vi "LDA_IP.vi"() -> (0 "error out":errorcluster)   [LabVIEW 2022 SP3]
uses:
  Globals/Meas_global.vi
  Globals/LDA_global.vi
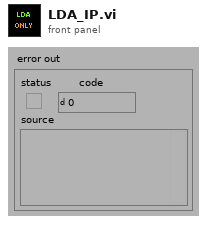
[diagram p1: front panel]
types:
  T1 = typedef "Setup.ctl" = enum16{"Run Program", "Show Setup", "Save Current Setup", "Setup Front Panel"}
  T2 = typedef "LDA_Channel.ctl" = cluster{"Wavelength (nm)":dbl, "Vel Comp":string, "Max Velocity":dbl, "Min Velocity":dbl, "Max Record length":u16, "Signal gain (dB)":i16, "High voltage":i16, "Optics Conversion Factor":dbl, "Min Record length":u16, "Multiply Velocity by -1":bool, "Signal to Noise Ratio":string, "Validation Ratio":string, "Probe":string, "Laser":string, "BSA":string, "Lense":string, "Beam Separation (mm)":dbl, "Focal Length (mm)":dbl, "COLOUR":u32, "BSA IP":string, "Velocity Range (m/s)":dbl, "Centre Velocity (m/s)":dbl, "Unshifted mW":dbl, "Shifted mW":dbl, "Bandwidth Hz":dbl, "Req Sampling Rate Hz":dbl, "Ch":i32, "CenterFreq Hz":dbl, "Laser IP":string, "Sync Delay (s)":dbl}
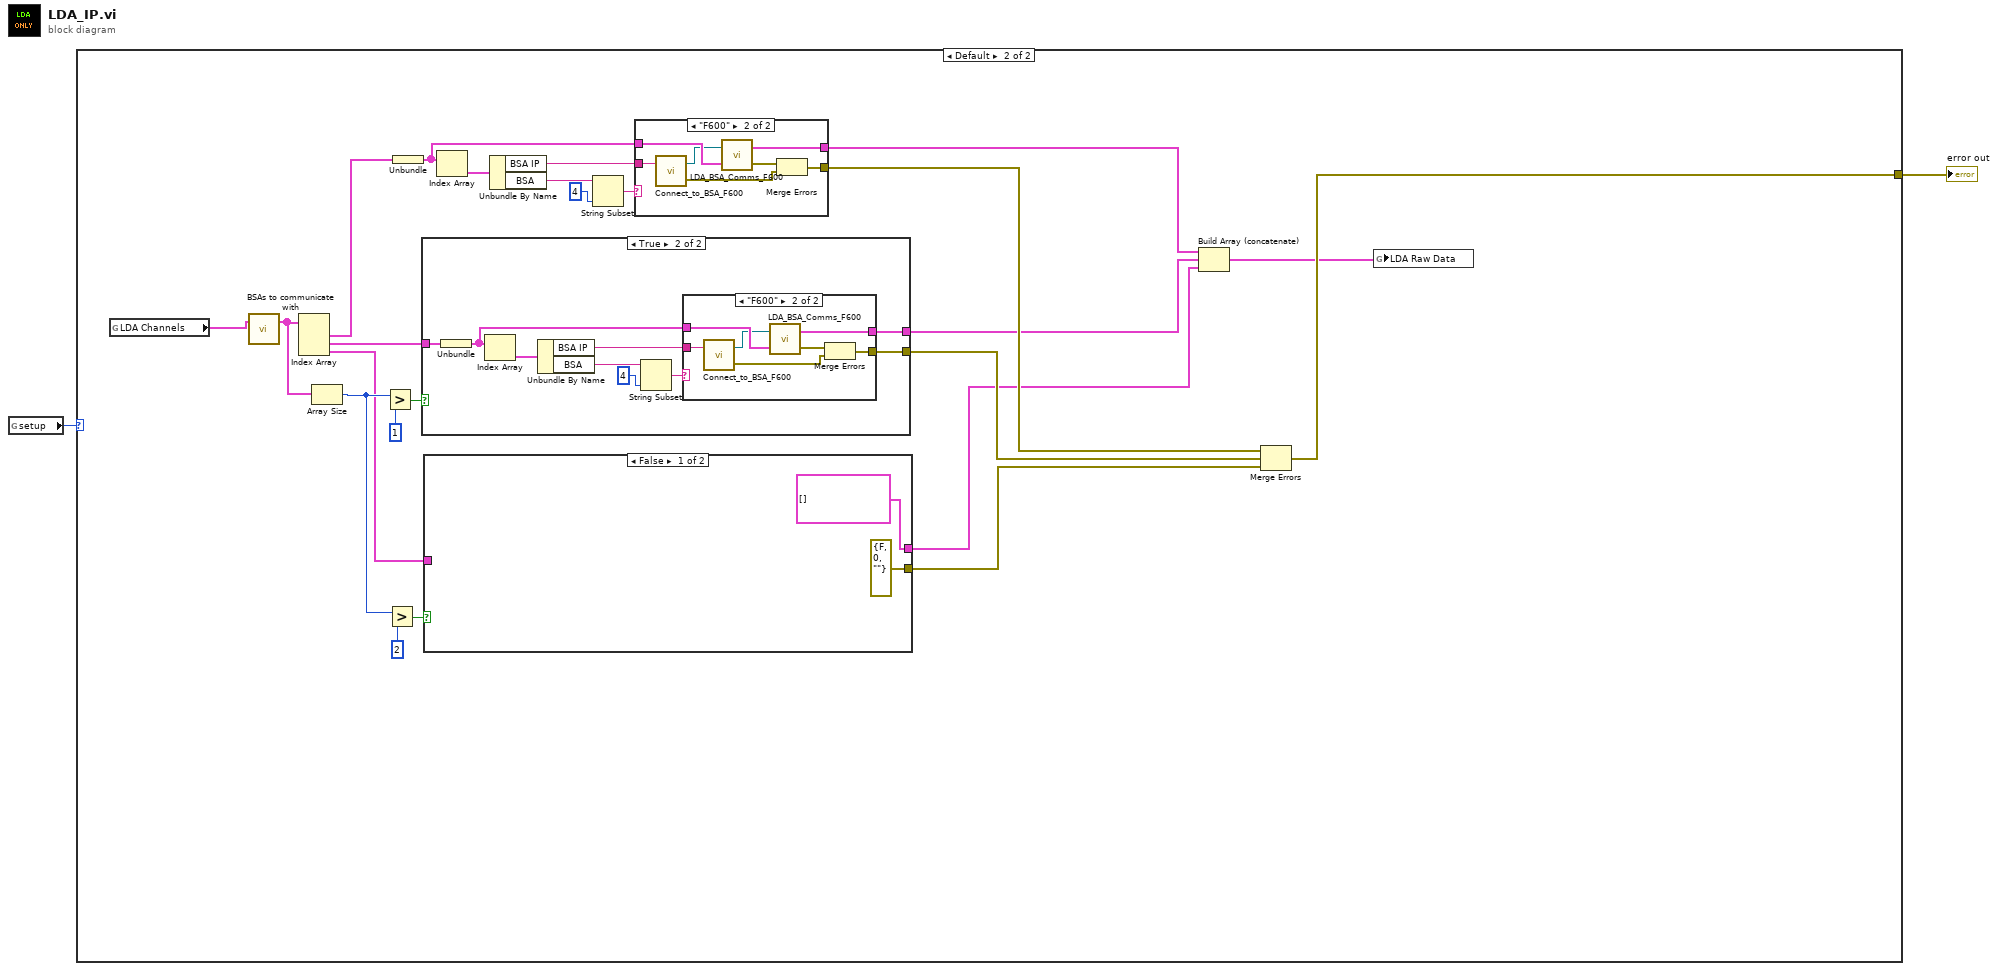
[diagram p0: block diagram]
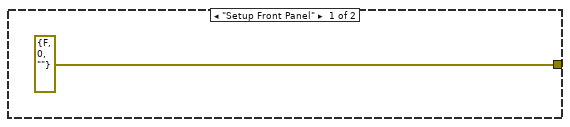
[diagram p2: hidden frame]
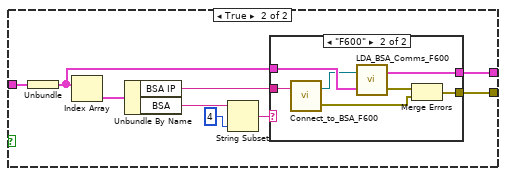
[diagram p3: hidden frame]
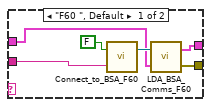
[diagram p4: hidden frame]
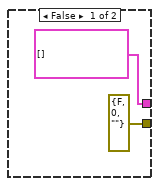
[diagram p5: hidden frame]
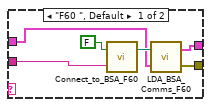
[diagram p6: hidden frame]
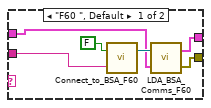
[diagram p7: hidden frame]
diagram:
  n1 = global read "Meas_global.vi" "setup"() -> (w1:T1)
  n2 = case shown="Default" w1 {
    tunnel: [errorcluster {"status"=FALSE, "code"=0, "source"=""} ("error out") w13] -> w2
    frame "Setup Front Panel" {
    }
    frame Default {
      n3 = global read "LDA_global.vi" "LDA Channels"() -> (w27:T2[])
      n4 = call "BSAs to communicate with.vi"("LDA Channels"=w27) -> ("BSAs to contact"=w18:cluster{T2[]}[])  [unwired: 2 in]
      n5 = Index Array(array=w18) -> (element #1=w26:cluster{T2[]}, element #2=w19:cluster{T2[]}, element #3=w6:cluster{T2[]})  [unwired: 3 in]
      n6 = Array Size(array=w18) -> (size(s)=w7:i32)
      n7 = Greater?(x=w7, y=1) -> (0:w16:bool)
      n8 = Greater?(x=w7, y=2) -> (0:w9:bool)
      n9 = Unbundle(w26) -> (w23:T2[])
      n10 = case shown="True" w16 {
        tunnel: w19 -> [_ w56]
        tunnel: [errorcluster {"status"=FALSE, "code"=0, "source"=""} ("error out") w55] -> w15
        tunnel: [cluster{dbl[][]}[] [] ("LDA Raw Data") w54] -> w11
        frame False {
        }
        frame True {
          n11 = Unbundle(w56) -> (w59:T2[])
          n12 = Index Array(array=w59) -> (element=w57:T2)  [unwired: 1 in]
          n13 = Unbundle By Name(w57) -> ("BSA IP"=w62:string, "BSA"=w60:string)
          n14 = String Subset(string=w60, length (rest)=4 ("length (rest)")) -> (substring=w61:string)  [unwired: 1 in]
          n15 = case shown="\"F600\"" w61 {
            tunnel: [w64 w69] -> w55
            tunnel: w59 -> [w67 w75]
            tunnel: w62 -> [w66 w73]
            tunnel: [w63 w74] -> w54
            frame "F60 ", Default {
              n16 = call "Connect_to_BSA_F60.vi"("BSA IP Number"=w66, "Force Reconnect"=FALSE) -> ("BSA"=w68:refnum<k7>)  [unwired: 1 out]
              n17 = call "LDA_BSA_Comms_F60.vi"("LDA Channels"=w67, "BSA"=w68) -> ("error out"=w64:errorcluster, "LDA Raw Data"=w63:cluster{dbl[][]}[])
            }
            frame "F600" {
              n18 = call "Connect_to_BSA_F600.vi"("BSA IP Number"=w73) -> ("error out"=w70:errorcluster, "F600"=w72:refnum<k7>)  [unwired: 1 in]
              n19 = call "LDA_BSA_Comms_F600.vi"("LDA Channels"=w75, "BSACtrl.IBSA F600"=w72) -> ("error out"=w71:errorcluster, "LDA Raw Data"=w74:cluster{dbl[][]}[])
              n20 = Merge Errors(w71, w70) -> (w69:errorcluster)
            }
          }
        }
      }
      n21 = case shown="False" w9 {
        tunnel: w6 -> [_ w32]
        tunnel: [errorcluster {"status"=FALSE, "code"=0, "source"=""} ("error out") w31] -> w4
        tunnel: [cluster{dbl[][]}[] [] ("LDA Raw Data") w30] -> w5
        frame False {
        }
        frame True {
          n22 = Unbundle(w32) -> (w35:T2[])
          n23 = Index Array(array=w35) -> (element=w33:T2)  [unwired: 1 in]
          n24 = Unbundle By Name(w33) -> ("BSA IP"=w38:string, "BSA"=w36:string)
          n25 = String Subset(string=w36, length (rest)=4 ("length (rest)")) -> (substring=w37:string)  [unwired: 1 in]
          n26 = case shown="\"F600\"" w37 {
            tunnel: [w40 w45] -> w31
            tunnel: w35 -> [w43 w51]
            tunnel: w38 -> [w42 w49]
            tunnel: [w39 w50] -> w30
            frame "F60 ", Default {
              n27 = call "Connect_to_BSA_F60.vi"("BSA IP Number"=w42, "Force Reconnect"=FALSE) -> ("BSA"=w44:refnum<k7>)  [unwired: 1 out]
              n28 = call "LDA_BSA_Comms_F60.vi"("LDA Channels"=w43, "BSA"=w44) -> ("error out"=w40:errorcluster, "LDA Raw Data"=w39:cluster{dbl[][]}[])
            }
            frame "F600" {
              n29 = call "Connect_to_BSA_F600.vi"("BSA IP Number"=w49) -> ("error out"=w46:errorcluster, "F600"=w48:refnum<k7>)  [unwired: 1 in]
              n30 = call "LDA_BSA_Comms_F600.vi"("LDA Channels"=w51, "BSACtrl.IBSA F600"=w48) -> ("error out"=w47:errorcluster, "LDA Raw Data"=w50:cluster{dbl[][]}[])
              n31 = Merge Errors(w47, w46) -> (w45:errorcluster)
            }
          }
        }
      }
      n32 = Index Array(array=w23) -> (element=w25:T2)  [unwired: 1 in]
      n33 = Unbundle By Name(w25) -> ("BSA IP"=w20:string, "BSA"=w22:string)
      n34 = String Subset(string=w22, length (rest)=4 ("length (rest)")) -> (substring=w21:string)  [unwired: 1 in]
      n35 = case shown="\"F600\"" w21 {
        tunnel: [w77 w82] -> w14
        tunnel: w23 -> [w80 w88]
        tunnel: w20 -> [w79 w86]
        tunnel: [w76 w87] -> w12
        frame "F60 ", Default {
          n36 = call "Connect_to_BSA_F60.vi"("BSA IP Number"=w79, "Force Reconnect"=FALSE) -> ("BSA"=w81:refnum<k7>)  [unwired: 1 out]
          n37 = call "LDA_BSA_Comms_F60.vi"("LDA Channels"=w80, "BSA"=w81) -> ("error out"=w77:errorcluster, "LDA Raw Data"=w76:cluster{dbl[][]}[])
        }
        frame "F600" {
          n38 = call "Connect_to_BSA_F600.vi"("BSA IP Number"=w86) -> ("error out"=w84:errorcluster, "F600"=w85:refnum<k7>)  [unwired: 1 in]
          n39 = call "LDA_BSA_Comms_F600.vi"("LDA Channels"=w88, "BSACtrl.IBSA F600"=w85) -> ("error out"=w83:errorcluster, "LDA Raw Data"=w87:cluster{dbl[][]}[])
          n40 = Merge Errors(w83, w84) -> (w82:errorcluster)
        }
      }
      n41 = Build Array (concatenate)(w12, w11, w5) -> (w10:cluster{dbl[][]}[])
      n42 = Merge Errors(w14, w15, w4) -> (w13:errorcluster)
      n43 = global write "LDA_global.vi" "LDA Raw Data"(w10) -> ()
    }
  }
  "error out" <- w2
